vi "Get Data Queue.vi"(8 "error in (no error)":errorcluster, 11 "Task Base in":refnum<class "Task Base.lvclass">) -> (0 "error out":errorcluster, 2 "Data Queue":refnum<queue>, 3 "Task Base out":refnum<class "Task Base.lvclass">)   [LabVIEW 2023, in "HAL GOOP4.lvlib" / "Task Base.lvclass"]
uses:
  Task Base.lvclass
  Task Base.lvclass/Task Base.ctl
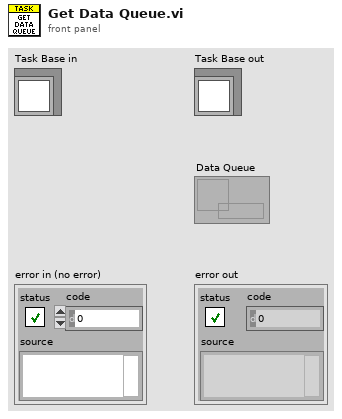
[diagram p1: front panel]
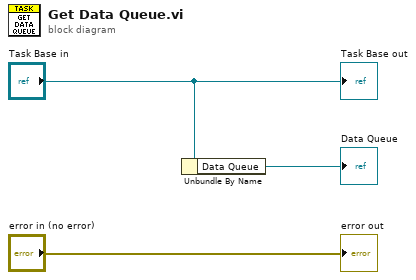
[diagram p0: block diagram]
diagram:
  n1 = Unbundle By Name("Task Base in") -> ("Data Queue"=→"Data Queue":refnum<queue>)
  "error out" <- "error in (no error)"
  "Task Base out" <- "Task Base in"
